vi "CelsiusToOthersFunction.vi"(0 "Celsius":dbl) -> (1 "k":dbl, 2 "f":dbl)   [LabVIEW 2020]
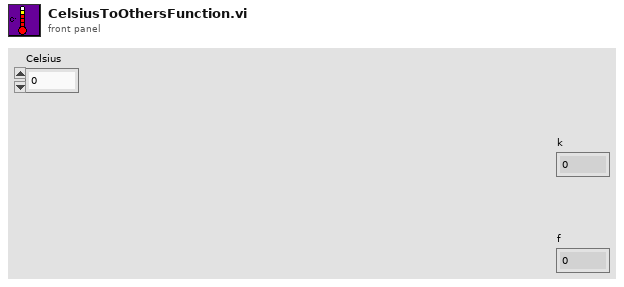
[diagram p1: front panel]
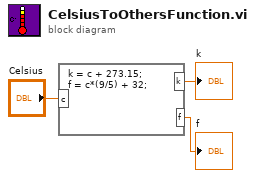
[diagram p0: block diagram]
diagram:
  n1 = formula code="k = c + 273.15;\nf = c*(9/5) + 32;"("c"="Celsius") -> ("k"=→"k":dbl, "f"=→"f":dbl)
